vi "Encoder trigger task-Generate data.vi"(8 "error in (no error)":errorcluster, 9 "Sample Clock Rate":dbl format="%#_6f", 10 "Number of samples in pockels modulation AO sequence":i32, 11 "Specified encoder trigger pulse width (us)":dbl) -> (0 "error":errorcluster, 1 "Number of samples in high pulse":i32, 2 "Encoder trigger data":dbl[](array[numeric]), 3 "Encoder trigger DO sequence":digitaldata, 4 "Sampling period (sec)":dbl format="%#_6f", 5 "# points in output waveform":i32, 6 "Pulse width (sec)":dbl format="%#_6f")   [LabVIEW 2020]
uses:
  <vilib>/GPower/Comparison/Library/IsOdd/IsOddI32.vi
  <vilib>/Waveform/DWDTOps.llb/Digital Pattern Generator (Single Value).vi
  <vilib>/Waveform/DWDTOps.llb/DWDT Append Digital Samples.vi
  <vilib>/GPower/Comparison/GPComparison.lvlib
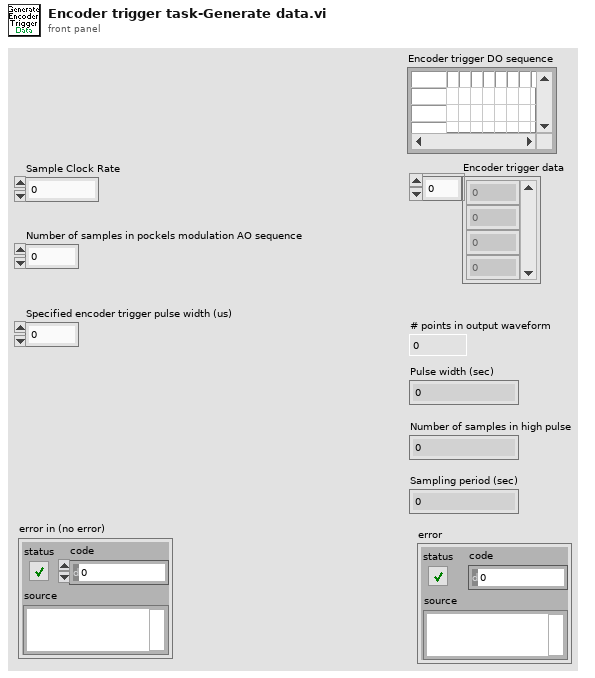
[diagram p1: front panel]
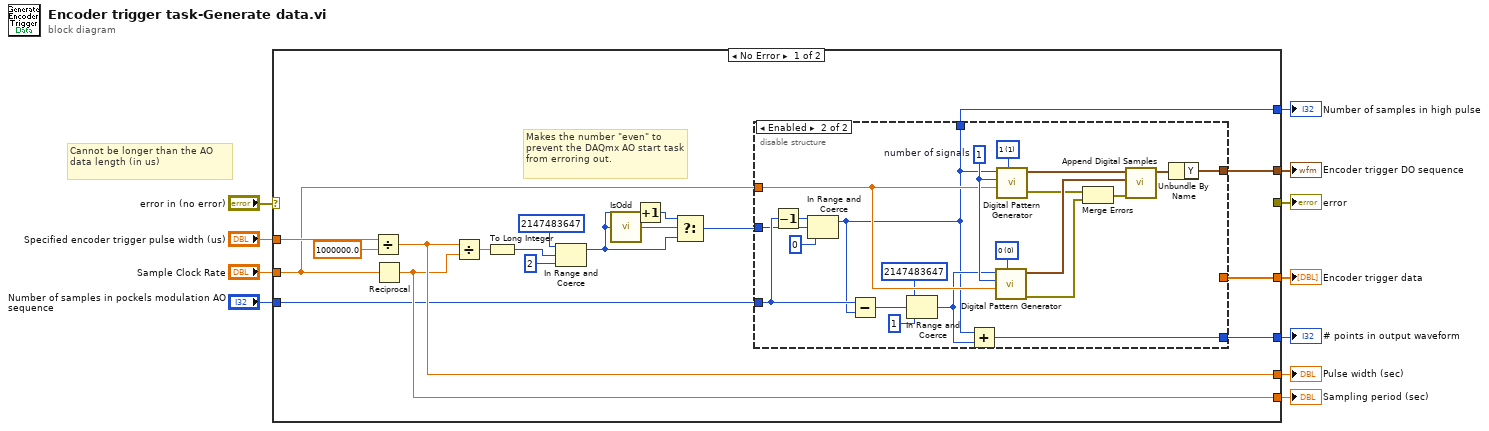
[diagram p0: block diagram]
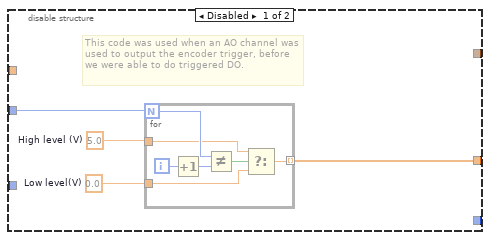
[diagram p2: hidden frame]
diagram:
  # "Cannot be longer than the AO data length (in us)"
  n1 = case shown="No Error" "error in (no error)" {
    selector: "error in (no error)" -> [_ w62]
    tunnel: [w29 _] -> w11
    tunnel: [_ w62] -> w10
    tunnel: "Specified encoder trigger pulse width (us)" -> [w28 _]
    tunnel: "Sample Clock Rate" -> [w17 _]
    tunnel: [w14 _] -> w6
    tunnel: [w27 _] -> w5
    tunnel: [w26 _] -> w4
    tunnel: [w16 _] -> w3
    tunnel: "Number of samples in pockels modulation AO sequence" -> [w12 _]
    tunnel: [w15 _] -> w1
    frame No Error {
      # "Makes the number \"even\" to prevent the DAQmx AO start task from erroring out."
      n2 = Divide(x=w28, y=1000000.0) -> (x/y=w27:dbl)
      n3 = Reciprocal(x=w17) -> (1/x=w26:dbl)
      n4 = Divide(x=w27, y=w26) -> (x/y=w18:dbl)
      n5 = To Long Integer(number=w18) -> (32bit integer=w19:i32)
      n6 = In Range and Coerce(upper limit=2147483647, x=w19, lower limit=2) -> (coerced(x)=w20:i32)  [unwired: 1 out]
      n7 = call-poly <vilib>:"IsOdd.vi"("x"=w20) -> ("Odd?"=w22:bool)  [unwired: 4 in]
      n8 = Increment(x=w20) -> (x+1=w21:i32)
      n9 = Select(t=w21, s=w22, f=w20) -> (s? t:f=w13:i32)
      n10 = disable-structure shown="Enabled" {
        disable-tunnel: [w33 _] -> w29
        disable-tunnel: w13 -> [w32 w43]
        disable-tunnel: w17 -> [_ w50]
        disable-tunnel: [_ w52] -> w16
        disable-tunnel: w12 -> [_ w45]
        disable-tunnel: [_ w51] -> w15
        disable-tunnel: [_ w41] -> w14
        frame Disabled {
          w30 = 5.0  # High level (V)
          w31 = 0.0  # Low level(V)
          # "This code was used when an AO channel was used to output the encoder trigger, before we were able to do triggered DO."
          n11 = for {
            N: w32 -> [w38]
            tunnel: w31 -> [w36]
            tunnel: w30 -> [w35]
            tunnel: [w34] -> w33 mode=indexing
            i -> [w40]
            n12 = Increment(x=w40) -> (x+1=w39:i32)
            n13 = Not Equal?(x=w38, y=w39) -> (x != y?=w37:bool)
            n14 = Select(t=w35, s=w37, f=w36) -> (s? t:f=w34:dbl)
          }
        }
        frame Enabled {
          w57 = u8 0 items=["0", "1", "Z", "L", "H", "X", "T", "V"] ("value")
          w58 = u8 1 items=["0", "1", "Z", "L", "H", "X", "T", "V"] ("value")
          w53 = u32 1  # number of signals
          n15 = Decrement(x=w45) -> (x-1=w42:i32)
          n16 = In Range and Coerce(upper limit=w42, x=w43, lower limit=0) -> (coerced(x)=w41:i32)  [unwired: 1 out]
          n17 = Subtract(x=w45, y=w41) -> (x-y=w48:i32)
          n18 = In Range and Coerce(upper limit=2147483647, x=w48, lower limit=1) -> (coerced(x)=w47:i32)  [unwired: 1 out]
          n19 = Add(x=w41, y=w47) -> (x+y=w52:i32)
          n20 = call-poly <vilib>:"Digital Pattern Generator.vi"("value"=w57, "sample rate"=w50, "number of signals"=w53, "number of samples"=w47) -> ("error out"=w56:errorcluster, "digital waveform"=w60:digitalwaveform)  [unwired: 1 in, 5 out]
          n21 = call-poly <vilib>:"Digital Pattern Generator.vi"("value"=w58, "sample rate"=w50, "number of signals"=w53, "number of samples"=w41) -> ("error out"=w55:errorcluster, "digital waveform"=w59:digitalwaveform)  [unwired: 1 in, 5 out]
          n22 = Merge Errors(w55, w56) -> (w54:errorcluster)
          n23 = call-poly <vilib>:"Append Digital Samples.vi"("error in (no error)"=w54, "digital waveform B"=w60, "digital waveform A"=w59) -> ("digital waveform out"=w61:digitalwaveform)  [unwired: 8 out]
          n24 = Unbundle By Name(w61) -> ("Y"=w51:digitaldata)
        }
      }
    }
    frame Error {
    }
  }
  "Encoder trigger data" <- w11
  "error" <- w10
  "Number of samples in high pulse" <- w6
  "Pulse width (sec)" <- w5
  "Sampling period (sec)" <- w4
  "# points in output waveform" <- w3
  "Encoder trigger DO sequence" <- w1
